vi "Do Action.vi"(8 "error in (no error)":errorcluster, 9 "Display Queue":refnum<queue>, 10 "tlc_User Event Reference.ctl":T1, 11 "Record in":refnum<class "Record.lvclass">) -> (0 "error out":errorcluster)   [LabVIEW 2010, in "Record.lvclass"]
doc: "Retrieve the cue that has been created by the Record Dialog Box and add it to the Cue List."
uses:
  Record.lvclass
  Controls/tlc_User Interface Command.ctl
  Controls/tlc_User Interface Data Type.ctl
  Controls/tlc_User Event Reference.ctl
  Record.lvclass/Record.ctl
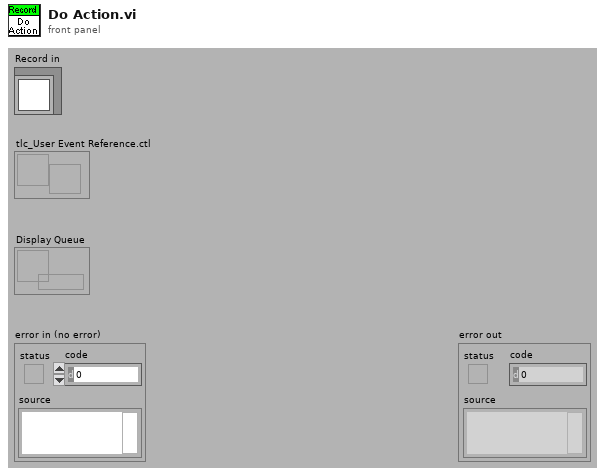
[diagram p1: front panel]
types:
  T1 = typedef "tlc_User Event Reference.ctl" = refnum<user-event>
  T2 = typedef "tlc_Cue_Information.ctl" = cluster{"Cue Name":string, "Wait Time (s)":u32, "Fade Time (s)":u32, "Follow Time (s)":u32, "Channels":T3[][]}
  T3 = typedef "channel.ctl" = cluster{"Intensity":dbl, " Color":u32, "Channel":i32}
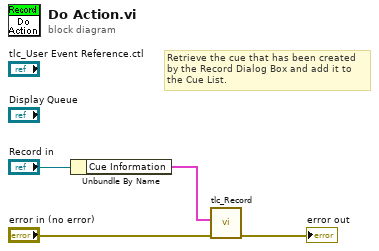
[diagram p0: block diagram]
diagram:
  # "Retrieve the cue that has been created by the Record Dialog Box and add it to the Cue List."
  n1 = Unbundle By Name "Unbundle By Name"("Record in") -> ("Cue Information"=w1:T2)
  n2 = call "tlc_Record.vi"("error in (no error)"="error in (no error)", "Cue"=w1) -> ("error out"=→"error out":errorcluster)  [unwired: 9 in]
